vi "Test.vi"   [LabVIEW 2017]
doc: "This VI is called when test mode begins, and will automatically be terminated when it ends. You can add manual or automatic tests and invoke them from the dashboard."
uses:
  5492_WPI_RobotDriveMotorSelectorEnum.ctl
  Public/Documents/Cross The Road Electronics/Phoenix-LabVIEW/Motor Controller/Controls/CTRE_Phoenix_MotorControl_FeedbackDevice.ctl
  Public/Documents/Cross The Road Electronics/Phoenix-LabVIEW/Motor Controller/Controls/CTRE_Phoenix_MotorControl_ControlMode.ctl
  <vilib>/Rock Robotics/WPI/Utilities/WPI_GetSetVariantRefNum.vi
  <vilib>/Rock Robotics/WPI/RobotDrive/WPI_RobotDriveSafetyCheck.vi
  Public/Documents/Cross The Road Electronics/Phoenix-LabVIEW/Motor Controller/Get/CTRE_Phoenix_MotorController_GetQuadratureData.vi
types:
  T1 = typedef "CTRE_Phoenix_MotorControl_ControlMode.ctl" = u16
  T2 = typedef "CTRE_Phoenix_MotorControl_FeedbackDevice.ctl" = i8
  T3 = typedef "5492_WPI_RobotDriveMotorSelectorEnum.ctl" = enum16{"Front left motor", "Front right motor", "Back left motor", "Back right motor"}
  T4 = typedef "WPI_RobotDriveDevRef.ctl" = cluster{"DevStatus":errorcluster, "Motors[]":T5[], "Square Inputs":bool, "Max Output":dbl}
  T5 = typedef "WPI_MotorControlDeviceRef.ctl" = cluster{"DeviceStatus":errorcluster, "Type":T6, "PWM":cluster{"PWM Channel":T7, "DeadBand":T8}, "CAN":cluster{"Device Number":u8, "SetOutput VI Ref":variant, "GetOutput VI Ref":variant, "Enable VI Ref":variant, "Disable VI Ref":variant, "Data":variant}, "Invert":bool, "DIO PWM":cluster{"PWM \"Enable\" Channel":T7, "DIOChannel":T9, "PWM Rate":dbl}}
  T6 = typedef "WPI_MotorControlType.ctl" = enum16{"PWM", "CAN", "DIO PWM"}
  T7 = typedef "FPGA_DIOPWMChannel.ctl" = enum8{"PWM 0", "PWM 1", "PWM 2", "PWM 3", "PWM 4", "PWM 5", "PWM 6", "PWM 7", "PWM 8", "PWM 9", "PWM MXP 0", "PWM MXP 1", "PWM MXP 2", "PWM MXP 3", "PWM MXP 4", "PWM MXP 5", "PWM MXP 6", "PWM MXP 7", "PWM MXP 8", "PWM MXP 9", "Invalid"}
  T8 = typedef "WPI_PWMDeadband.ctl" = cluster{"Name":string, "maxPositivePwm":i32, "minPositivePwm":i32, "centerPwm":i32, "maxNegativePwm":i32, "minNegativePwm":i32, "angularRange":u16}
  T9 = typedef "FPGA_DIOChannel.ctl" = enum8{"DIO 0", "DIO 1", "DIO 2", "DIO 3", "DIO 4", "DIO 5", "DIO 6", "DIO 7", "DIO 8", "DIO 9", "DIO MXP 0", "DIO MXP 1", "DIO MXP 2", "DIO MXP 3", "DIO MXP 4", "DIO MXP 5", "DIO MXP 6", "DIO MXP 7", "DIO MXP 8", "DIO MXP 9", "DIO MXP 10", "DIO MXP 11", "DIO MXP 12", "DIO MXP 13", "DIO MXP 14", "DIO MXP 15", "SPI Port CS1", "SPI Port CS2", "SPI Port CS3", "SPI Port MISO", "SPI Port MOSI", "Invalid"}
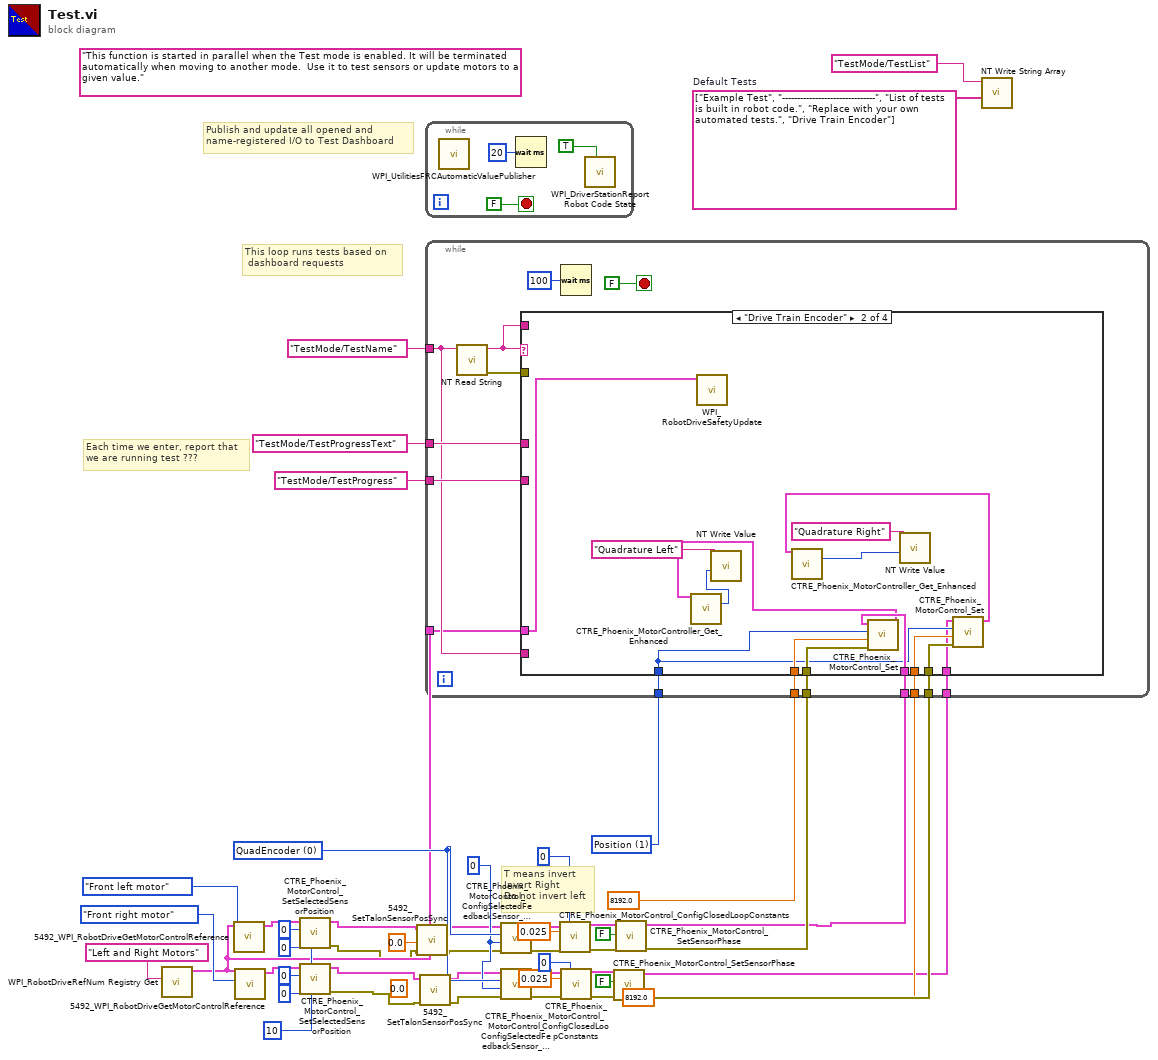
[diagram p0: block diagram]
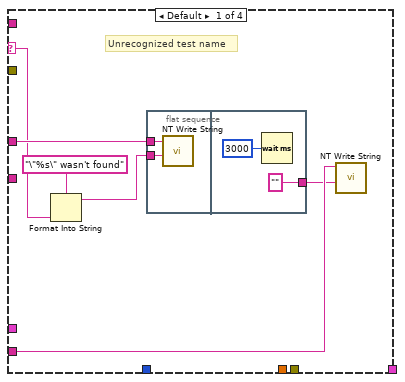
[diagram p2: hidden frame]
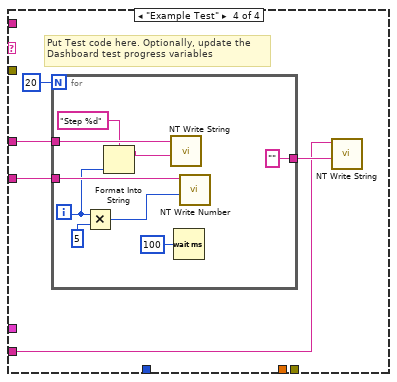
[diagram p4: hidden frame]
diagram:
  w18 = u32 10 ("timeoutMs")
  w15 = T1 1 items=["PercentOutput"=0, "Position"=1, "Velocity"=2, "Current"=3, "Follower"=5, "MotionProfile"=6, "MotionMagic"=7, "MotionMagicArc"=8, "MotionProfileArc"=10, "Disabled"=15] ("Control Mode")
  (unwired) 0.0 ("Output")
  w39 = 0 ("pidLoopIdx")
  w40 = T2 0 items=["None"=-1, "QuadEncoder"=0, "Analog"=2, "Tachometer"=4, "Pulse Width Encoded Position"=8, "Sensor Sum (S0 + S1)"=9, "Sensor Difference (D0 - D1)"=10, "Remote Source 0"=11, "Remote Source 1"=12, "Software Emulated"=15] ("Feedback Device")
  w45 = string[] ["Example Test", "-------------------------------", "List of tests is built in robot code.", "Replace with your own automated tests.", "Drive Train Encoder"]  # Default Tests
  (unwired) "This function is started in parallel when the Test mode is enabled. It will be terminated automatically when moving to another mode.  Use it to test sensors or update motors to a given value."
  # "T means invert\nInvert Right\nDo not invert left"
  # "This loop runs tests based on \n dashboard requests"
  # "Publish and update all opened and\nname-registered I/O to Test Dashboard"
  # "Each time we enter, report that\nwe are running test ???"
  n1 = call <vilib>:"WPI_RobotDriveRefNum Registry Get.vi"("refnum name"="Left and Right Motors") -> ("RobotDriveDevRef"=w12:T4)  [unwired: 1 in, 9 out]
  n2 = call "5492_WPI_RobotDriveGetMotorControlReference.vi"("MotorIndex"=5492_WPI_RobotDriveMotorSelectorEnum."Front left motor", "RobotDriveDevRef"=w12) -> ("MotorControlDeviceRef"=w24:T5)  [unwired: 9 out]
  n3 = call "5492_WPI_RobotDriveGetMotorControlReference.vi"("MotorIndex"=5492_WPI_RobotDriveMotorSelectorEnum."Front right motor", "RobotDriveDevRef"=w12) -> ("MotorControlDeviceRef"=w21:T5)  [unwired: 9 out]
  n4 = call "CTRE_Phoenix_MotorControl_SetSelectedSensorPosition.vi"("timeoutMs"=w18, "pidLoopIdx"=u32 0, "New Sensor Position"=0, "PhoenixMotorControlDevRef"=w24) -> ("error out"=w5:errorcluster, "PhoenixMotorControlDevRef"=w10:T5)  [unwired: 6 in]
  n5 = call "CTRE_Phoenix_MotorControl_SetSelectedSensorPosition.vi"("timeoutMs"=w18, "pidLoopIdx"=u32 0, "New Sensor Position"=0, "PhoenixMotorControlDevRef"=w21) -> ("error out"=w4:errorcluster, "PhoenixMotorControlDevRef"=w8:T5)  [unwired: 6 in]
  n6 = call "5492_SetTalonSensorPosSync.vi"("error in (no error)"=w5, "Pos"=0.0 ("Output"), "CAN Talon SRX Ref In"=w10) -> ("error out"=w6:errorcluster, "CAN Talon SRX Ref Out"=w9:T5)  [unwired: 7 in]
  n7 = call "5492_SetTalonSensorPosSync.vi"("error in (no error)"=w4, "CAN Talon SRX Ref In"=w8) -> ("error out"=w3:errorcluster, "CAN Talon SRX Ref Out"=w7:T5)  [unwired: 8 in]
  n8 = while {
    stop <- FALSE stop-if-true
    n9 = call <vilib>:"WPI_UtilitiesFRCAutomaticValuePublisher.vi"() -> ()  [unwired: 12 in]
    n10 = Wait (ms)(milliseconds to wait=u32 20) -> ()  [unwired: 1 out]
    n11 = call <vilib>:"WPI_DriverStationReport Robot Code State.vi"("Test"=TRUE ("Autonomous")) -> ()  [unwired: 10 in, 1 out]
  }
  n12 = call "CTRE_Phoenix_MotorControl_ConfigSelectedFeedbackSensor_Enhanced.vi"("error in (no error)"=w6, "pidLoopIdx"=w39, "Feedback Device"=w40, "PhoenixMotorControlDevRef"=w9) -> ("error out"=w37:errorcluster, "PhoenixMotorControlDevRef"=w38:T5)  [unwired: 6 in]
  n13 = call "CTRE_Phoenix_MotorControl_ConfigSelectedFeedbackSensor_Enhanced.vi"("error in (no error)"=w3, "pidLoopIdx"=w39, "Feedback Device"=w40, "PhoenixMotorControlDevRef"=w7) -> ("error out"=w35:errorcluster, "PhoenixMotorControlDevRef"=w36:T5)  [unwired: 6 in]
  n14 = call "CTRE_Phoenix_MotorControl_ConfigClosedLoopConstants.vi"("PhoenixMotorControlDevRef"=w38, "slotIdx"=0, "P"=0.025, "error in (no error)"=w37) -> ("PhoenixMotorControlDevRef"=w32:T5, "error out"=w31:errorcluster)  [unwired: 10 in]
  n15 = call "CTRE_Phoenix_MotorControl_ConfigClosedLoopConstants.vi"("PhoenixMotorControlDevRef"=w36, "slotIdx"=0, "P"=0.025, "error in (no error)"=w35) -> ("PhoenixMotorControlDevRef"=w33:T5, "error out"=w34:errorcluster)  [unwired: 10 in]
  n16 = call "CTRE_Phoenix_MotorControl_SetSensorPhase.vi"("error in (no error)"=w34, "PhaseSensor"=FALSE, "PhoenixMotorControlDevRef"=w33) -> ("error out"=w14:errorcluster, "PhoenixMotorControlDevRef"=w1:T5)  [unwired: 7 in]
  n17 = call "CTRE_Phoenix_MotorControl_SetSensorPhase.vi"("error in (no error)"=w31, "PhaseSensor"=FALSE, "PhoenixMotorControlDevRef"=w32) -> ("error out"=w17:errorcluster, "PhoenixMotorControlDevRef"=w2:T5)  [unwired: 7 in]
  n18 = while {
    tunnel: "TestMode/TestName" ("Name") -> [w61]
    tunnel: "TestMode/TestProgressText" ("Name") -> [w64]
    tunnel: "TestMode/TestProgress" ("Name") -> [w63]
    tunnel: w17 -> [w59]
    tunnel: 8192.0 ("Output") -> [w58]
    tunnel: w15 -> [w57]
    tunnel: w2 -> [w56]
    tunnel: w14 -> [w55]
    tunnel: 8192.0 ("Output") -> [w54]
    tunnel: w1 -> [w53]
    tunnel: w12 -> [w52]
    stop <- FALSE stop-if-true
    n19 = call <vilib>:"NT Read String.vi"("Name"=w61) -> ("error out"=w60:errorcluster, "String"=w62:string)  [unwired: 9 in]
    n20 = case shown="\"Drive Train Encoder\"" w62 {
      selector: w62 -> [w71 _ _ _]
      tunnel: w61 -> [w68 _ _ w91]
      tunnel: w64 -> [w72 _ _ w94]
      tunnel: w63 -> [_ _ _ w95]
      tunnel: w62 -> [_ _ _ _]
      tunnel: w60 -> [_ _ _ _]
      tunnel: w59 -> [_ w86 _ _]
      tunnel: w58 -> [_ w85 _ _]
      tunnel: w57 -> [_ w80 _ _]
      tunnel: w56 -> [_ w84 _ _]
      tunnel: w55 -> [_ w82 _ _]
      tunnel: w54 -> [_ w81 _ _]
      tunnel: w53 -> [_ w79 _ _]
      tunnel: w52 -> [_ w77 _ _]
      frame Default {
        # "Unrecognized test name"
        n21 = Format Into String(format string="\"%s\" wasn't found" ("Name"), w71) -> (resulting string=w70:string)  [unwired: 2 in, 1 out]
        n22 = flat-sequence {
          tunnel: w72 -> [w73]
          tunnel: w70 -> [w74]
          tunnel: ["" ("Name")] -> w67
          frame #0 {
            n23 = call <vilib>:"NT Write String.vi"("String"=w74, "Name"=w73) -> ()  [unwired: 9 in, 1 out]
          }
          frame #1 {
            n24 = Wait (ms)(milliseconds to wait=u32 3000) -> ()  [unwired: 1 out]
          }
        }
        n25 = call <vilib>:"NT Write String.vi"("String"=w67, "Name"=w68) -> ()  [unwired: 9 in, 1 out]
      }
      frame "Drive Train Encoder" {
        n26 = call <vilib>:"WPI_RobotDriveSafetyUpdate.vi"("RobotDriveDevRef"=w77) -> ()  [unwired: 1 in, 10 out]
        n27 = call "CTRE_Phoenix_MotorControl_Set.vi"("error in (no error)"=w86, "Output"=w85, "Control Mode"=w80, "PhoenixMotorControlDevRef"=w84) -> ("PhoenixMotorControlDevRef"=w83:T5)  [unwired: 6 in, 1 out]
        n28 = call-poly "CTRE_Phoenix_MotorController_Get_Enhanced.vi"("PhoenixMotorControlDevRef"=w83) -> ("Quadrature Position"=w88:i32)  [unwired: 11 in, 3 out]
        n29 = call-poly <vilib>:"NT Write Value.vi"("Numeric"=w88, "Name"="Quadrature Left") -> ()  [unwired: 9 in, 1 out]
        n30 = call "CTRE_Phoenix_MotorControl_Set.vi"("error in (no error)"=w82, "Output"=w81, "Control Mode"=w80, "PhoenixMotorControlDevRef"=w79) -> ("PhoenixMotorControlDevRef"=w78:T5)  [unwired: 6 in, 1 out]
        n31 = call-poly "CTRE_Phoenix_MotorController_Get_Enhanced.vi"("PhoenixMotorControlDevRef"=w78) -> ("Quadrature Position"=w87:i32)  [unwired: 11 in, 3 out]
        n32 = call-poly <vilib>:"NT Write Value.vi"("Numeric"=w87, "Name"="Quadrature Right") -> ()  [unwired: 9 in, 1 out]
      }
      frame "" {
        # "No test to run"
      }
      frame "Example Test" {
        # "Put Test code here. Optionally, update the\nDashboard test progress variables"
        n33 = for {
          N: 20 -> [_]
          tunnel: w95 -> [w104]
          tunnel: w94 -> [w102]
          tunnel: ["" ("String")] -> w92
          i -> [w99]
          n34 = Multiply(x=w99, y=u32 5 ("milliseconds to wait")) -> (x*y=w100:u32)
          n35 = Format Into String(format string="Step %d", w99) -> (resulting string=w97:string)  [unwired: 2 in, 1 out]
          n36 = call <vilib>:"NT Write String.vi"("String"=w97, "Name"=w102) -> ()  [unwired: 9 in, 1 out]
          n37 = Wait (ms)(milliseconds to wait=u32 100) -> ()  [unwired: 1 out]
          n38 = call <vilib>:"NT Write Number.vi"("Numeric"=w100, "Name"=w104) -> ()  [unwired: 9 in, 1 out]
        }
        n39 = call <vilib>:"NT Write String.vi"("String"=w92, "Name"=w91) -> ()  [unwired: 9 in, 1 out]
      }
    }
    n40 = Wait (ms)(milliseconds to wait=u32 100) -> ()  [unwired: 1 out]
  }
  n41 = call <vilib>:"NT Write String Array.vi"("String Array"=w45, "Name"="TestMode/TestList") -> ()  [unwired: 9 in, 1 out]
